vi "Cal Time If Fit.vi"(8 "error in (no error)":errorcluster, 9 "CurWeek(0)":i32, 10 "StandardStartTime":timestamp, 11 "Source Time(\"\")":string) -> (0 "error out":errorcluster, 2 "Fit(False)":bool)   [LabVIEW 2015, in "Admin_Actor.lvlib" / "CalAttendance.lvclass"]
uses:
  CalAttendance/CalAttendance.lvclass
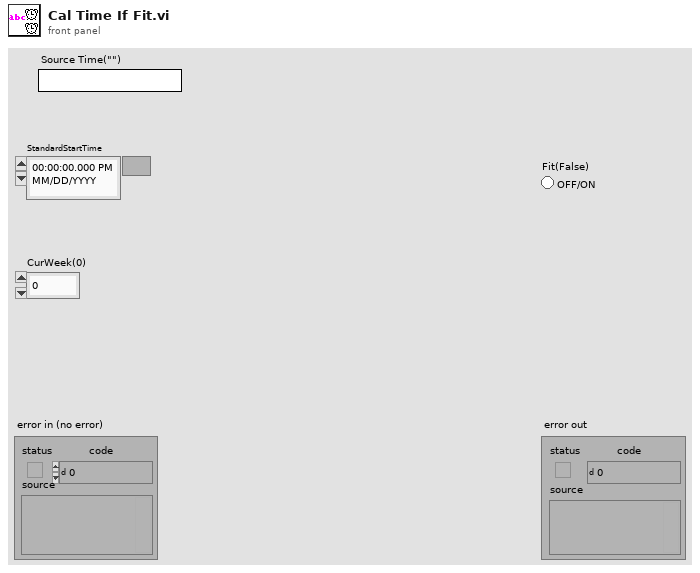
[diagram p1: front panel]
types:
  T1 = typedef "LVDateTimeRec.ctl" = cluster{"fractional second":dbl, "second":i32, "minute":i32, "hour":i32, "day of month":i32, "month":i32, "year":i32, "day of week":i32, "day of year":i32, "DST":i32}
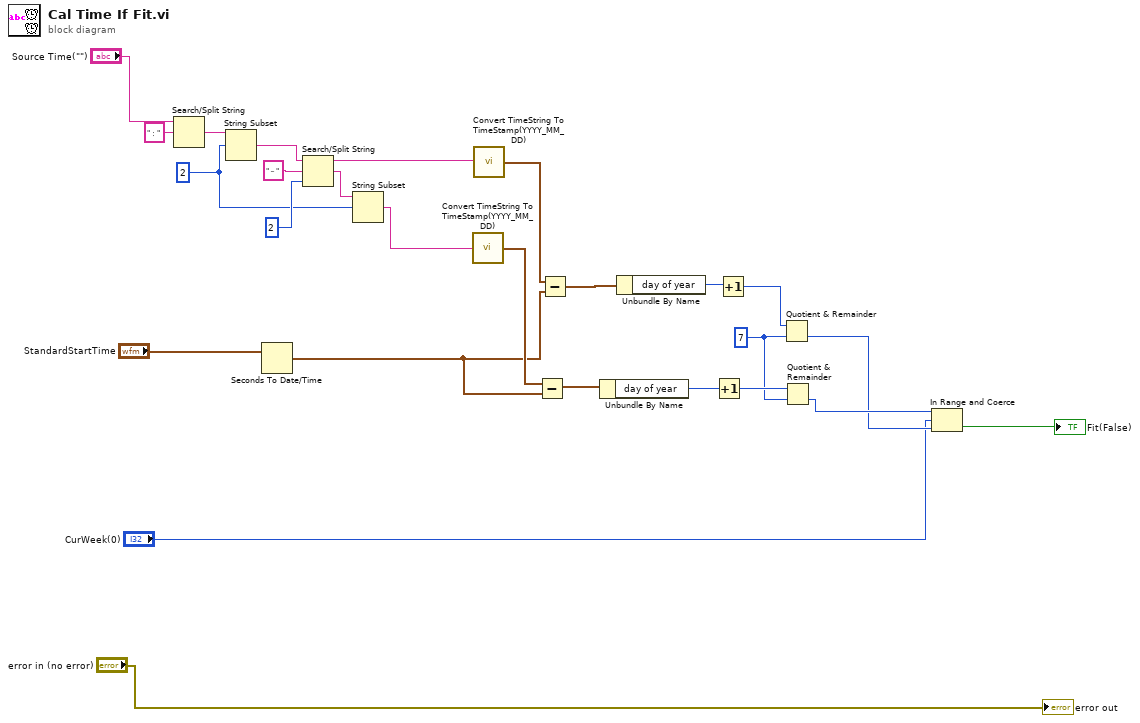
[diagram p0: block diagram]
diagram:
  w6 = 7 ("y")
  w18 = 2 ("offset (0)")
  n1 = Search/Split String(string="Source Time(\"\")", search string/char (-)="：") -> (match + rest of string=w21:string)  [unwired: 1 in, 2 out]
  n2 = String Subset(string=w21, offset (0)=w18) -> (substring=w20:string)  [unwired: 1 in]
  n3 = Seconds To Date/Time(time stamp (now)="StandardStartTime") -> (date time rec=w13:T1)  [unwired: 1 in]
  n4 = Search/Split String(string=w20, search string/char (-)="～", offset (0)=2) -> (substring before match=w22:string, match + rest of string=w19:string)  [unwired: 1 out]
  n5 = String Subset(string=w19, offset (0)=w18) -> (substring=w17:string)  [unwired: 1 in]
  n6 = call "Convert TimeString To TimeStamp(YYYY_MM_DD).vi"("时间字符串（H:MM）"=w17) -> ("date time rec"=w14:T1)
  n7 = call "Convert TimeString To TimeStamp(YYYY_MM_DD).vi"("时间字符串（H:MM）"=w22) -> ("date time rec"=w16:T1)
  n8 = Subtract(x=w14, y=w13) -> (x-y=w11:T1)
  n9 = Subtract(x=w16, y=w13) -> (x-y=w12:T1)
  n10 = Unbundle By Name(w11) -> ("day of year"=w8:i32)
  n11 = Unbundle By Name(w12) -> ("day of year"=w10:i32)
  n12 = Increment(x=w8) -> (x+1=w7:i32)
  n13 = Increment(x=w10) -> (x+1=w9:i32)
  n14 = Quotient & Remainder(x=w9, y=w6) -> (floor(x/y)=w4:i32)  [unwired: 1 out]
  n15 = Quotient & Remainder(x=w7, y=w6) -> (floor(x/y)=w5:i32)  [unwired: 1 out]
  n16 = In Range and Coerce(upper limit=w5, x="CurWeek(0)", lower limit=w4) -> (In Range?=→"Fit(False)":bool)  [unwired: 1 out]
  "error out" <- "error in (no error)"
